vi "Run VI Analyzer.vi"(8 "error in":errorcluster, 9 "File ID":i32=-1, 10 "Commit ID":i32=-1, 11 "Peer Review in":refnum<class "Peer Review.lvclass">) -> (0 "error out":errorcluster, 3 "Peer Review out":refnum<class "Peer Review.lvclass">)   [LabVIEW 2020, in "Peer Review.lvclass"]
uses:
  Peer Review.lvclass
  Peer Review.lvclass/Peer Review.ctl
  user32.dll
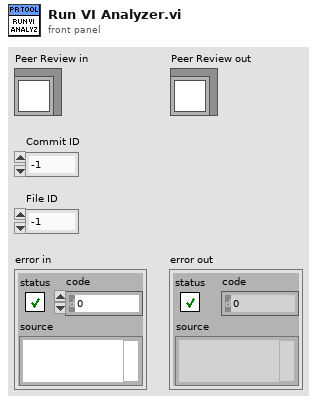
[diagram p1: front panel]
types:
  T1 = typedef "Peer Review.lvclass/File Info.ctl" = cluster{"File ID":i32, "Commit ID":i32, "Reviewed Hash":string, "Relative Path":string, "File Path":path, "File Checksum":string, "State":T2, "FP Changes":i32, "BD Changes":i32, "FP Bounds Error":dbl, "BD Bounds Error":dbl, "Lines Added":i32, "Lines Removed":i32, "Analysis Passes":i32, "Analysis Fails":i32, "Attribute Changes":i32, "Reentrancy State":string, "Cyclomatic Complexity":i32, "Node Count":i32, "Revision Number":u32, "LabVIEW Version":string, "Description":string, "Master Path":path, "Master Checksum":string, "VI Type":T3, "LabVIEW File":bool, "Review Complete":bool, "File Ref":refnum<vi>}
  T2 = typedef "Peer Review.lvclass/File State.ctl" = enum16{"Interrogation Needed", "Modified", "Deleted", "Added", "Matches Previous", "No Changes", "Moved"}
  T3 = typedef "Peer Review.lvclass/VI Type.ctl" = enum32{"invalid VI type", "Standard VI", "Control VI", "Global VI", "Polymorphic VI", "Configuration VI", "SubSystem", "Facade VI", "Method VI", "Statechart Diagram VI"}
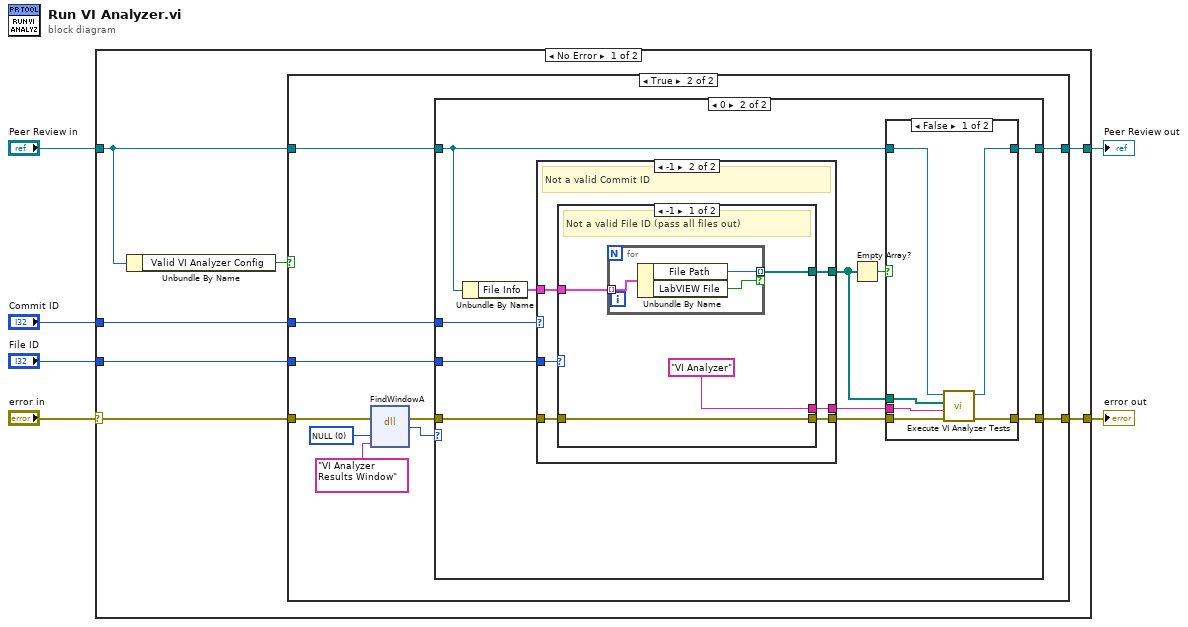
[diagram p0: block diagram]
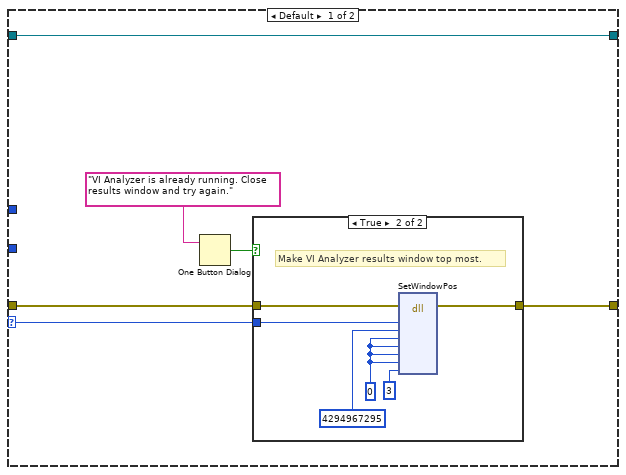
[diagram p3: hidden frame]
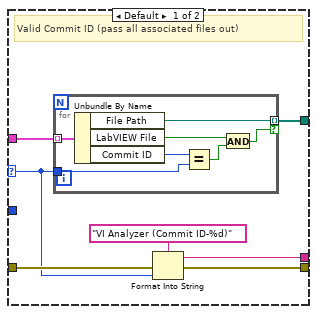
[diagram p5: hidden frame]
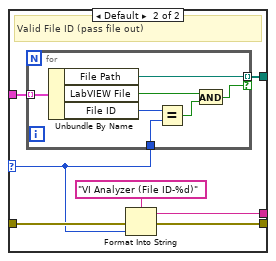
[diagram p6: hidden frame]
diagram:
  n1 = case shown="No Error" "error in" {
    selector: "error in" -> [w9 w99]
    tunnel: "Peer Review in" -> [w8 w100]
    tunnel: "Commit ID" -> [w12 _]
    tunnel: [w13 w99] -> w3
    tunnel: [w10 w100] -> w2
    tunnel: "File ID" -> [w11 _]
    frame No Error {
      n2 = Unbundle By Name(w8) -> ("Valid VI Analyzer Config"=w7:bool)
      n3 = case shown="True" w7 {
        tunnel: [w14 w25] -> w13
        tunnel: w12 -> [_ w24]
        tunnel: w11 -> [_ w23]
        tunnel: [w15 w22] -> w10
        tunnel: w9 -> [w14 w21]
        tunnel: w8 -> [w15 w16]
        frame False {
        }
        frame True {
          w20 = 0 items=["NULL"]
          n4 = dll-call lib="user32.dll" fn="FindWindowA" label="FindWindow"(error in=w21, "lpszClassName"=w20, "lpszWindowName"="VI Analyzer Results Window") -> (error out=w18:errorcluster, "hWnd"=w17:u32)  [unwired: 4 in, 1 out]
          n5 = case shown="0" w17 {
            selector: w17 -> [w29 _]
            tunnel: [w26 w49] -> w25
            tunnel: w24 -> [_ w45]
            tunnel: w23 -> [_ w44]
            tunnel: [w31 w43] -> w22
            tunnel: w16 -> [w31 w42]
            tunnel: w18 -> [w27 w40]
            frame Default {
              n6 = One Button Dialog(message="VI Analyzer is already running. Close results window and try again.") -> (true=w28:bool)  [unwired: 1 in]
              n7 = case shown="True" w28 {
                tunnel: w29 -> [_ w35]
                tunnel: w27 -> [w32 w34]
                tunnel: [w32 w33] -> w26
                frame False {
                }
                frame True {
                  w38 = 0
                  # "Make VI Analyzer results window top most."
                  n8 = dll-call lib="USER32.DLL" fn="SetWindowPos"(error in=w34, "hWnd"=w35, "hWndInsertAfter"=u32 4294967295 ("x-y"), "left"=w38, "top"=w38, "width"=w38, "height"=w38, "fuFlags"=u32 3 ("x .or. y?")) -> (error out=w33:errorcluster)  [unwired: 8 in, 3 out]
                }
              }
            }
            frame 0 {
              n9 = Unbundle By Name(w42) -> ("File Info"=w48:T1[])
              n10 = case shown="-1" w45 {
                selector: w45 -> [w53 _]
                tunnel: w48 -> [w56 w69]
                tunnel: [w55 w68] -> w46
                tunnel: w44 -> [_ w67]
                tunnel: w40 -> [w54 w66]
                tunnel: [w51 w65] -> w41
                tunnel: [w50 w64] -> w39
                frame Default {
                  # "Valid Commit ID (pass all associated files out)"
                  n11 = for {
                    tunnel: w56 -> [w63] mode=indexing
                    tunnel: w53 -> [w62]
                    tunnel: [w61] -> w55 mode=indexing if=w58
                    n12 = Unbundle By Name(w63) -> ("File Path"=w61:path, "LabVIEW File"=w59:bool, "Commit ID"=w60:i32)
                    n13 = Equal?(x=w60, y=w62) -> (x = y?=w57:bool)
                    n14 = And(x=w59, y=w57) -> (x .and. y?=w58:bool)
                  }
                  n15 = Format Into String(format string="VI Analyzer (Commit ID-%d)", error in=w54, w53) -> (resulting string=w50:string, error out=w51:errorcluster)  [unwired: 1 in]
                }
                frame -1 {
                  # "Not a valid Commit ID"
                  n16 = case shown="-1" w67 {
                    selector: w67 -> [_ w78]
                    tunnel: w69 -> [w73 w83]
                    tunnel: [w72 w82] -> w68
                    tunnel: w66 -> [w71 w80]
                    tunnel: [w71 w79] -> w65
                    tunnel: ["VI Analyzer" w77] -> w64
                    frame -1 {
                      # "Not a valid File ID (pass all files out)"
                      n17 = for {
                        tunnel: w73 -> [w76] mode=indexing
                        tunnel: [w75] -> w72 mode=indexing if=w74
                        n18 = Unbundle By Name(w76) -> ("File Path"=w75:path, "LabVIEW File"=w74:bool)
                      }
                    }
                    frame Default {
                      # "Valid File ID (pass file out)"
                      n19 = for {
                        tunnel: w83 -> [w90] mode=indexing
                        tunnel: [w89] -> w82 mode=indexing if=w87
                        tunnel: w78 -> [w85]
                        n20 = Unbundle By Name(w90) -> ("File Path"=w89:path, "LabVIEW File"=w88:bool, "File ID"=w84:i32)
                        n21 = Equal?(x=w84, y=w85) -> (x = y?=w86:bool)
                        n22 = And(x=w88, y=w86) -> (x .and. y?=w87:bool)
                      }
                      n23 = Format Into String(format string="VI Analyzer (File ID-%d)", error in=w80, w78) -> (resulting string=w77:string, error out=w79:errorcluster)  [unwired: 1 in]
                    }
                  }
                }
              }
              n24 = Empty Array?(array=w46) -> (empty?=w47:bool)
              n25 = case shown="False" w47 {
                tunnel: w41 -> [w95 w98]
                tunnel: [w91 w98] -> w49
                tunnel: w46 -> [w96 _]
                tunnel: [w93 w97] -> w43
                tunnel: w42 -> [w92 w97]
                tunnel: w39 -> [w94 _]
                frame False {
                  n26 = call "Execute VI Analyzer Tests.vi"("error in"=w95, "File Name"=w94, "File List"=w96, "Peer Review in"=w92) -> ("error out"=w91:errorcluster, "Peer Review out"=w93:refnum<class "Peer Review.lvclass">)  [unwired: 6 in]
                }
                frame True {
                }
              }
            }
          }
        }
      }
    }
    frame Error {
    }
  }
  "error out" <- w3
  "Peer Review out" <- w2
